vi "Get Slope and Offset.vi"(8 "raw max":sgl, 9 "raw min":sgl, 10 "emin":sgl, 11 "emax":sgl) -> (2 "c":sgl, 3 "m":sgl)   [LabVIEW 2018]
panel:
  out "x+y":sgl
  out "error out":errorcluster
  in  "error in (no error)":errorcluster
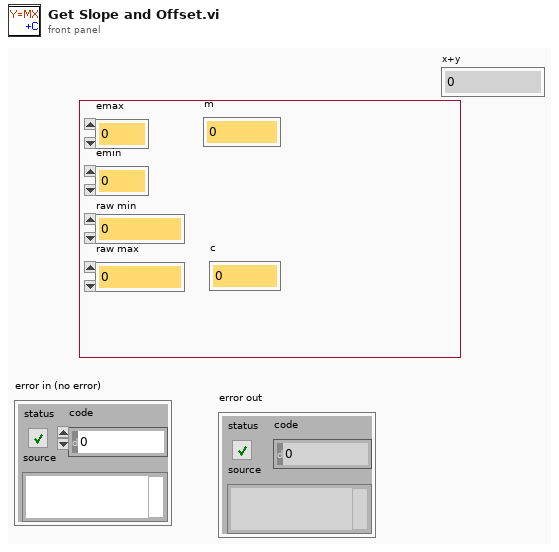
[diagram p1: front panel]
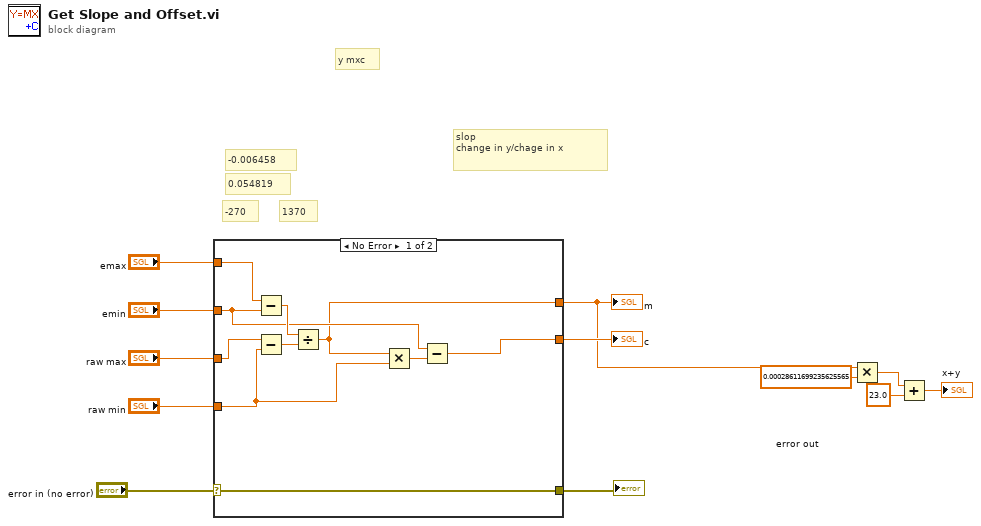
[diagram p0: block diagram]
diagram:
  # "y mxc"
  # "slop \nchange in y/chage in x"
  # "1370"
  # "-270"
  # "0.054819"
  # "-0.006458"
  n1 = case shown="No Error" "error in (no error)" {
    selector: "error in (no error)" -> [w18 w23]
    tunnel: "emin" -> [w17 _]
    tunnel: "raw min" -> [w16 _]
    tunnel: "emax" -> [w15 _]
    tunnel: "raw max" -> [w13 _]
    tunnel: [w14 _] -> w5
    tunnel: [w19 _] -> w8
    tunnel: [w18 w23] -> w6
    frame No Error {
      n2 = Subtract(x=w15, y=w17) -> (x-y=w22:sgl)
      n3 = Subtract(x=w13, y=w16) -> (x-y=w21:sgl)
      n4 = Divide(x=w22, y=w21) -> (x/y=w14:sgl)
      n5 = Multiply(x=w14, y=w16) -> (x*y=w20:sgl)
      n6 = Subtract(x=w17, y=w20) -> (x-y=w19:sgl)
    }
    frame Error {
    }
  }
  "error out" <- w6
  "m" <- w5
  "c" <- w8
  n7 = Multiply(x=w5, y=sgl 0.000286117) -> (x*y=w3:sgl)
  n8 = Add(x=w3, y=sgl 23.0) -> (x+y=→"x+y":sgl)
